vi "Configure the LCD display.vi"(5 "Enable to Query":bool, 7 "Enable to Setup":bool, 8 "error in":errorcluster, 9 "Sets the brightness":u8(ring)=1 items=["bright"=2, "drak"=1], 10 "Sets the contrast":u8(ring)=1 items=["8"=8, "7"=7, "6"=6, "5"=5, "4"=4, "3"=3, "2"=2, "1"=1], 11 "VISA resource name":refnum<visa-resource-name>) -> (0 "error out":errorcluster, 1 "Query the brightness":string, 2 "Query the contrast":string, 3 "VISA resource name out":refnum<visa-resource-name>)   [LabVIEW 2011, in "GPT-9000.lvlib"]
uses:
  <instrlib>/GPT-9000/GPT-9000.lvlib
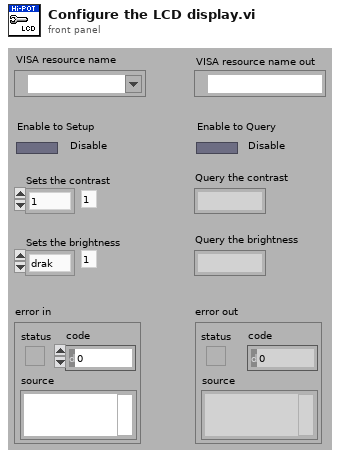
[diagram p1: front panel]
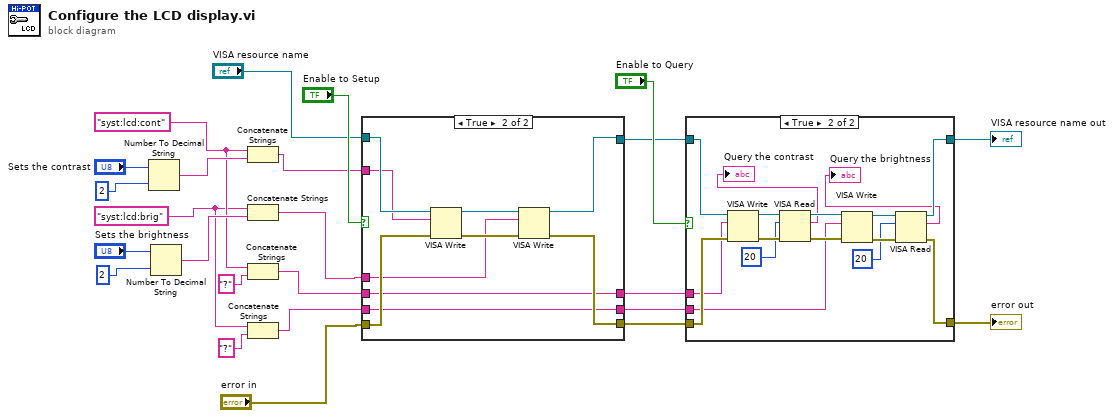
[diagram p0: block diagram]
diagram:
  w10 = "syst:lcd:brig"
  w11 = "syst:lcd:cont"
  n1 = Number To Decimal String(number="Sets the contrast", width (-)=i16 2) -> (decimal integer string=w20:string)
  n2 = Number To Decimal String(number="Sets the brightness", width (-)=i16 2) -> (decimal integer string=w19:string)
  n3 = Concatenate Strings(w11, w20) -> (w17:string)
  n4 = Concatenate Strings(w10, w19) -> (w16:string)
  n5 = Concatenate Strings(w11, "?" ("string")) -> (w4:string)
  n6 = Concatenate Strings(w10, "?" ("string")) -> (w3:string)
  n7 = case shown="True" "Enable to Setup" {
    tunnel: w17 -> [_ w36]
    tunnel: w16 -> [_ w33]
    tunnel: "VISA resource name" -> [w28 w37]
    tunnel: "error in" -> [w27 w38]
    tunnel: [w28 w32] -> w13
    tunnel: [w27 w31] -> w12
    tunnel: w4 -> [w26 w30]
    tunnel: w3 -> [w25 w29]
    tunnel: [w26 w30] -> w2
    tunnel: [w25 w29] -> w1
    frame False {
    }
    frame True {
      n8 = VISA Write(VISA resource name=w37, write buffer=w36, error in (no error)=w38) -> (VISA resource name out=w35:refnum<visa-resource-name>, error out=w34:errorcluster)  [unwired: 1 out]
      n9 = VISA Write(VISA resource name=w35, write buffer=w33, error in (no error)=w34) -> (VISA resource name out=w32:refnum<visa-resource-name>, error out=w31:errorcluster)  [unwired: 1 out]
    }
  }
  n10 = case shown="True" "Enable to Query" {
    tunnel: w13 -> [w40 w56]
    tunnel: w12 -> [w39 w55]
    tunnel: [w40 w44] -> w6
    tunnel: [w39 w43] -> w5
    tunnel: w2 -> [_ w54]
    tunnel: w1 -> [_ w48]
    frame False {
    }
    frame True {
      n11 = VISA Write(VISA resource name=w56, write buffer=w54, error in (no error)=w55) -> (VISA resource name out=w52:refnum<visa-resource-name>, error out=w53:errorcluster)  [unwired: 1 out]
      n12 = VISA Read(VISA resource name=w52, byte count=u32 20, error in (no error)=w53) -> (VISA resource name out=w50:refnum<visa-resource-name>, read buffer=→"Query the contrast":string, error out=w49:errorcluster)  [unwired: 1 out]
      n13 = VISA Write(VISA resource name=w50, write buffer=w48, error in (no error)=w49) -> (VISA resource name out=w46:refnum<visa-resource-name>, error out=w47:errorcluster)  [unwired: 1 out]
      n14 = VISA Read(VISA resource name=w46, byte count=u32 20, error in (no error)=w47) -> (VISA resource name out=w44:refnum<visa-resource-name>, read buffer=→"Query the brightness":string, error out=w43:errorcluster)  [unwired: 1 out]
    }
  }
  "VISA resource name out" <- w6
  "error out" <- w5
